vi "WPI_CameraGet Color Enable.vi"(8 "error in (no error)":errorcluster, 11 "CameraDevRef":T1={"Camera Address"="192.168.0.90", "CameraStatus"={"status"=FALSE, "code"=0, "source"=""}}) -> (0 "error out":errorcluster, 2 "Color Enabled":bool, 3 "CameraDevRef Out":T1)   [LabVIEW 2017]
doc: "Returns whether the the image from the camera will be encoded in color, or just in grayscale. Grayscale images are smaller in size and may simplify processing in some circumstances.\n\nThis software is licensed. Open the labview\\readme\\WPI Robotics Library Open Source License.txt file for more information."
uses:
  <vilib>/Rock Robotics/WPI/Camera/WPI_CameraDevRef.ctl
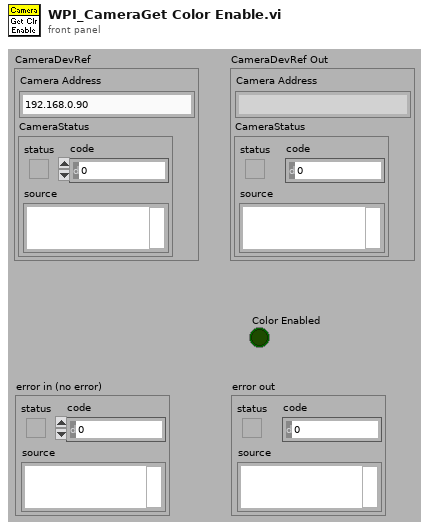
[diagram p1: front panel]
types:
  T1 = typedef "WPI_CameraDevRef.ctl" = cluster{"Camera Address":string, "CameraStatus":errorcluster}
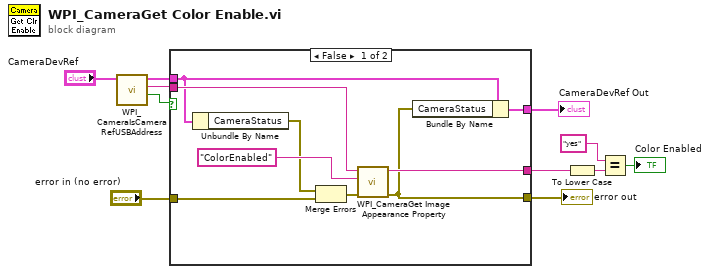
[diagram p0: block diagram]
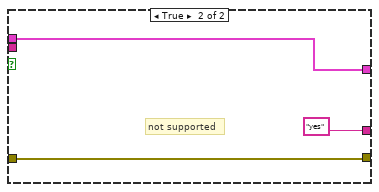
[diagram p2: hidden frame]
diagram:
  n1 = call <vilib>:"WPI_CameraIsCameraRefUSBAddress.vi"("CameraDevRef"="CameraDevRef") -> ("USB?"=w1:bool, "Camera Address Out"=w2:string, "CameraDevRef out"=w3:T1)  [unwired: 7 in, 1 out]
  n2 = case shown="False" w1 {
    tunnel: w2 -> [w19 _]
    tunnel: "error in (no error)" -> [w18 w21]
    tunnel: [w16 "yes"] -> w10
    tunnel: w3 -> [w12 w23]
    tunnel: [w15 w23] -> w6
    tunnel: [w14 w21] -> w5
    frame False {
      n3 = Unbundle By Name(w12) -> ("CameraStatus"=w13:errorcluster)
      n4 = Merge Errors(w13, w18) -> (w17:errorcluster)
      n5 = call <vilib>:"WPI_CameraGet Image Appearance Property.vi"("error in (no error)"=w17, "Prop String"="ColorEnabled" ("Property Name"), "address"=w19) -> ("error out"=w14:errorcluster, "Value"=w16:string)  [unwired: 1 in, 6 out]
      n6 = Bundle By Name(cluster=w12, "CameraStatus"=w14) -> (w15:T1)
    }
    frame True {
      # "not supported"
    }
  }
  "CameraDevRef Out" <- w6
  "error out" <- w5
  n7 = To Lower Case(string=w10) -> (all lower case string=w9:string)
  n8 = Equal?(x="yes", y=w9) -> (x = y?=→"Color Enabled":bool)
